vi "Compare 2 Icons.vi"(8 "error in (no error)":errorcluster, 11 "VI Reference":refnum<vi>) -> (0 "error out":errorcluster, 2 "Cycle time (For debug)":dbl, 3 "Match?":bool)   [LabVIEW 2021]
uses:
  <vilib>/LabVIEW Icon API/lv_icon/Controls/LabVIEW Icon Stored Information.ctl
  <vilib>/LabVIEW Icon API/lv_icon/Classes/Layer/Layer.lvclass
  <vilib>/LabVIEW Icon API/lv_icon/Controls/BodyText.ctl
  <vilib>/LabVIEW Icon API/lv_icon/Controls/Font.ctl
  <vilib>/LabVIEW Icon API/lv_icon/Controls/Alignment.ctl
  <vilib>/LabVIEW Icon API/lv_icon/Classes/Icon/Icon.lvclass
  <vilib>/LabVIEW Icon API/LabVIEW Icon API.lvlib
  <vilib>/LabVIEW Icon API/lv_icon/lv_icon.lvlib
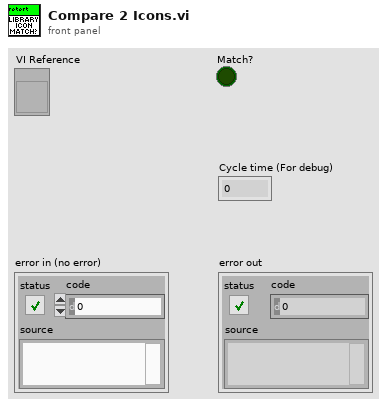
[diagram p1: front panel]
types:
  T1 = typedef "LabVIEW Icon Stored Information.ctl" = cluster{"Text Visible?":bool, "Text Opacity":u8, "Templ Visible?":bool, "Templ Opacity":u8, "Relative Path from 1 to 2":path, "Image":picture, "All User Layers":refnum<class "Layer.lvclass">[], "Body Text":T2}
  T2 = typedef "BodyText.ctl" = cluster{"Line 1 text":string, "Line 2 text":string, "Line 3 text":string, "Line 4 text":string, "Line 1 color":u32, "Line 2 color":u32, "Line 3 color":u32, "Line 4 color":u32, "Body Text Spec":cluster{"Font":T3, "Alignment":T4, "Size":u8}, "Center text vertically":bool, "Capitalize Text":bool}
  T3 = typedef "Font.ctl" = string
  T4 = typedef "Alignment.ctl" = u16
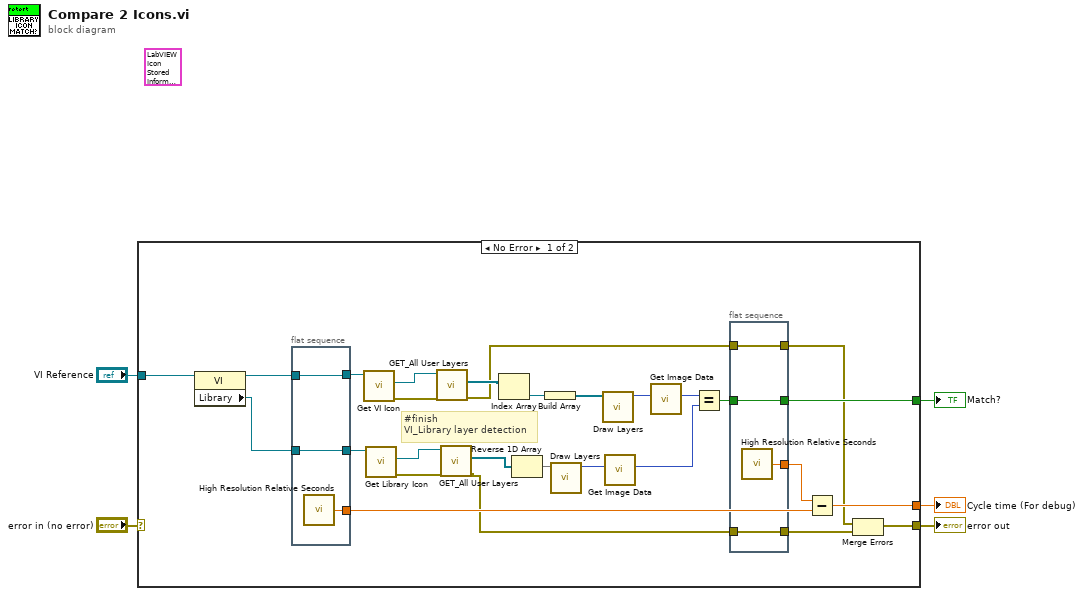
[diagram p0: block diagram]
diagram:
  (unwired) T1 {"Text Visible?"=TRUE, "Text Opacity"=100, "Templ Visible?"=TRUE, "Templ Opacity"=100, "Relative Path from 1 to 2"=path "", "Image"=bytes[0], "All User Layers"=[refnum, refnum, refnum], "Body Text"={"Line 1 text"="", "Line 2 text"="", "Line 3 text"="", "Line 4 text"="", "Line 1 color"=0, "Line 2 color"=0, "Line 3 color"=0, "Line 4 color"=0, "Body Text Spec"={"Font"="", "Alignment"=0, "Size"=0}, "Center text vertically"=FALSE, "Capitalize Text"=FALSE}} ("Icon Data")
  n1 = case shown="No Error" "error in (no error)" {
    selector: "error in (no error)" -> [_ w41]
    tunnel: [w23 _] -> w5
    tunnel: [w20 _] -> w4
    tunnel: "VI Reference" -> [w8 _]
    tunnel: [w10 w41] -> w1
    frame No Error {
      # "#finish\nVI_Library layer detection"
      n2 = property class="VI"(reference=w8) -> (reference out=w7:refnum<vi>, "Library"=w6:refnum<vi>)  [unwired: 1 in, 1 out]
      n3 = flat-sequence {
        tunnel: w7 -> [w40]
        tunnel: [w40] -> w25
        tunnel: [w39] -> w21
        tunnel: w6 -> [w38]
        tunnel: [w38] -> w9
        frame #0 {
          n4 = call <vilib>:"High Resolution Relative Seconds.vi"() -> ("relative seconds"=w39:dbl)
        }
      }
      n5 = call <vilib>:"Get VI Icon.vi"("VI Refnum in"=w25) -> ("error out"=w15:errorcluster, "Icon"=w32:refnum<class "Icon.lvclass">)  [unwired: 8 in, 1 out]
      n6 = call <vilib>:"Get Library Icon.vi"("Library Refnum in"=w9) -> ("error out"=w28:errorcluster, "Icon"=w29:refnum<class "Icon.lvclass">)  [unwired: 8 in, 1 out]
      n7 = call-dynamic "GET_All User Layers.vi"("error in (no error)"=w15, "Icon.lvclass in"=w32) -> ("error out"=w14:errorcluster, "User Layer"=w33:refnum<class "Layer.lvclass">[])  [unwired: 7 in, 1 out]
      n8 = call-dynamic "GET_All User Layers.vi"("error in (no error)"=w28, "Icon.lvclass in"=w29) -> ("error out"=w13:errorcluster, "User Layer"=w26:refnum<class "Layer.lvclass">[])  [unwired: 7 in, 1 out]
      n9 = Index Array(array=w33) -> (element=w31:refnum<class "Layer.lvclass">)  [unwired: 1 in]
      n10 = Reverse 1D Array(array=w26) -> (reversed array=w18:refnum<class "Layer.lvclass">[])
      n11 = Build Array(w31) -> (w19:refnum<class "Layer.lvclass">[])
      n12 = call <vilib>:"Draw Layers.vi"("Layers"=w18) -> ("Picture"=w17:picture)  [unwired: 4 in, 6 out]
      n13 = call <vilib>:"Draw Layers.vi"("Layers"=w19) -> ("Picture"=w16:picture)  [unwired: 4 in, 6 out]
      n14 = call <vilib>:"Get Image Data.vi"("Pic In"=w17) -> ("Pic Out"=w27:picture)  [unwired: 2 in, 8 out]
      n15 = call <vilib>:"Get Image Data.vi"("Pic In"=w16) -> ("Pic Out"=w30:picture)  [unwired: 2 in, 8 out]
      n16 = Equal?(x=w30, y=w27) -> (x = y?=w24:bool)
      n17 = flat-sequence {
        tunnel: w24 -> [w37]
        tunnel: [w37] -> w23
        tunnel: [w36] -> w22
        tunnel: w14 -> [w35]
        tunnel: w13 -> [w34]
        tunnel: [w35] -> w11
        tunnel: [w34] -> w12
        frame #0 {
          n18 = call <vilib>:"High Resolution Relative Seconds.vi"() -> ("relative seconds"=w36:dbl)
        }
      }
      n19 = Subtract(x=w22, y=w21) -> (x-y=w20:dbl)
      n20 = Merge Errors(w11, w12) -> (w10:errorcluster)
    }
    frame Error {
    }
  }
  "Match?" <- w5
  "Cycle time (For debug)" <- w4
  "error out" <- w1
